vi "SetupTest.vi"(11 "Python version":string="3.9") -> ()   [LabVIEW 2020]
panel:
  in  "stop":bool
  out "Console":string
  in  "Raspberry Pi":T1={"IP Address"="raspberrypi.local", "Username"="pi", "password"="raspberry"}
  # "1. Mac Users - you might have to install commandline tools by typing xcode-select --install into the terminal and saying \"ok\"\n2. Now install paramiko - sudo -H pip3 install paramiko --ignore-installed\n3. Now install scp - sudo pip3 install scp\n4. Getting the IP address and setting up the SDCard\n     1.  https://www.raspberrypi.org/documentation/configuration/wireless/headless.md - get it on the WiFi\n     2.  https://www.raspberrypi.org/documentation/remote-access/ssh/README.md - step 3 for headless - enable SSH\n     3. https://www.raspberrypi.org/documentation/remote-access/ip-address.md to get IP address\n     3. https://www.raspberrypi.org/documentation/remote-access/ssh/unix.md - test out ssh\n5. Ping it  - ping raspberrypi.local - that will give you the IP Address\n6. SSH in\n7. Change your password"
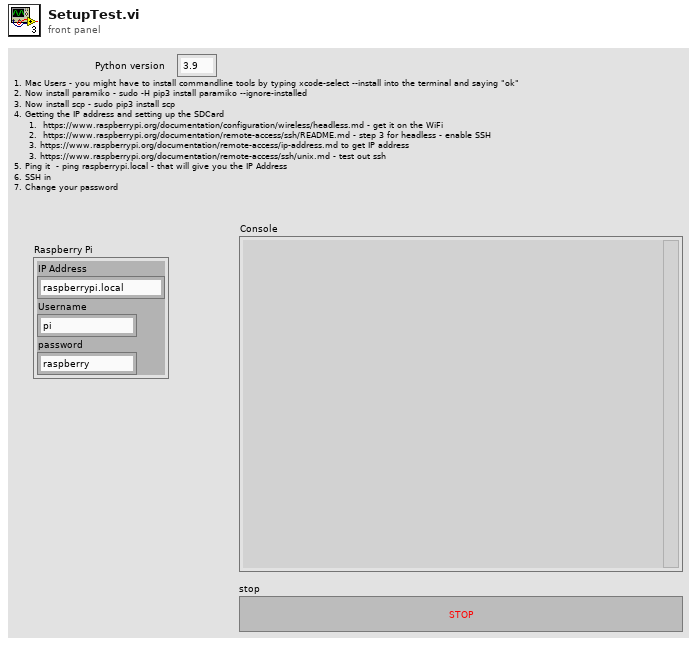
[diagram p1: front panel]
types:
  T1 = cluster{"IP Address":string, "Username":string, "password":string}
  T2 = typedef "PythonCtrl.ctl" = cluster{"session":refnum<k35>, "PyPath":path}
  T3 = typedef "eventvkey.ctl" = enum16{"ASCII", "Enter", "Return", "Shift", "Ctrl", "Alt", "Cmd", "Opt", "Caps", "NumLock", "Clear", "Break", "Up", "Down", "Left", "Right", "Insert", "Delete", "Home", "End", "PageUp", "PageDown", "Escape", "Help", "Pause", "ScrollLock", "F1", "F2", "F3", "F4", "F5", "F6", "F7", "F8", "F9", "F10", "F11", "F12", "F13", "F14", "F15", "F16", "F17", "F18", "F19", "F20", "F21", "F22", "F23", "F24", "Play", "VolumeUp", "VolumeDown", "Mute", "Two Byte Char"}
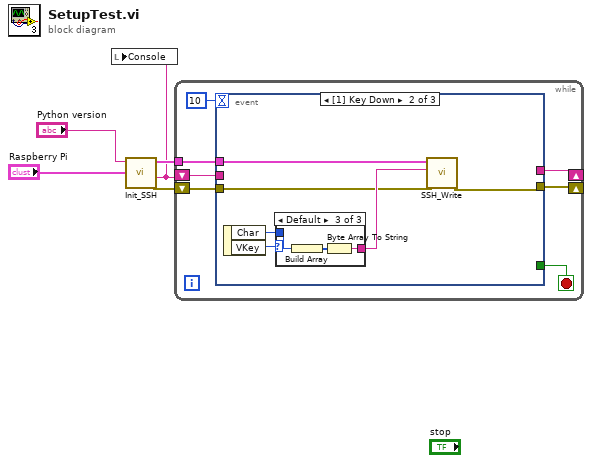
[diagram p0: block diagram]
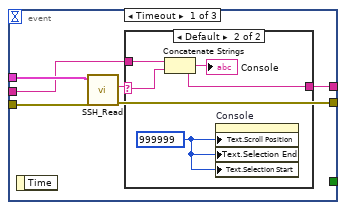
[diagram p2: hidden frame]
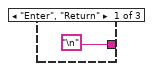
[diagram p4: hidden frame]
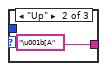
[diagram p5: hidden frame]
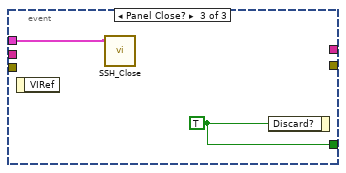
[diagram p6: hidden frame]
diagram:
  n1 = call "Init_SSH.vi"("Raspberry Pi"="Raspberry Pi", "Python version"="Python version") -> ("error out"=w2:errorcluster, "Console out"=w1:string, "Python"=w3:T2)  [unwired: 7 in]
  n2 = local write "Console"(w1) -> ()
  n3 = while {
    tunnel: w3 -> [w11]
    shift-right: [w8] -> _
    shift-left: w1 -> [w6]
    shift-right: [w7] -> _
    shift-left: w2 -> [w9]
    stop <- w12 stop-if-true
    n4 = event shown="[1] Key Down" {
      selector: _ -> [_ _ _]
      dyn-events: _ -> [_ _ _]
      timeout: 10 -> [_ _ _]
      tunnel: [_ _ w36] -> w12
      tunnel: w11 -> [w18 w27 w35]
      tunnel: w9 -> [w17 w25 _]
      tunnel: [w14 _ _] -> w8
      tunnel: [w16 w24 _] -> w7
      tunnel: w6 -> [w15 _ _]
      event Timeout {
        n5 = event-data() -> ()  [unwired: 1 in, 1 out]
        n6 = call "SSH_Read.vi"("error in (no error)"=w17, "Python"=w18) -> ("error out"=w16:errorcluster, "Reply"=w13:string)  [unwired: 7 in, 1 out]
        n7 = case shown="Default" w13 {
          selector: w13 -> [_ w20]
          tunnel: w15 -> [w19 w23]
          tunnel: [w19 w22] -> w14
          frame "" {
          }
          frame Default {
            w21 = u32 999999 ("Text.Scroll Position")
            n8 = Concatenate Strings(w23, w20) -> (w22:string)
            "Console" <- w22
            n9 = property on="Console" class="Str"("Text.Scroll Position"=w21, "Text.Selection End"=w21, "Text.Selection Start"=w21) -> ()  [unwired: 2 in, 2 out]
          }
        }
      }
      event Key Down {
        n10 = event-data() -> ("Char"=w29:i16, "VKey"=w28:T3)  [unwired: 1 in]
        n11 = case shown="Default" w28 {
          tunnel: w29 -> [_ _ w34]
          tunnel: ["\n" ("replace string (\"\")") "\u001b[A" ("replace string (\"\")") w32] -> w26
          frame "Enter", "Return" {
          }
          frame "Up" {
          }
          frame Default {
            n12 = Build Array(w34) -> (w33:i16[])
            n13 = Byte Array To String(unsigned byte array=w33) -> (string=w32:string)
          }
        }
        n14 = call "SSH_Write.vi"("error in (no error)"=w25, "Text to write"=w26, "Python in"=w27) -> ("error out"=w24:errorcluster)  [unwired: 7 in, 1 out]
      }
      event Panel Close? {
        w36 = TRUE ("Discard?")
        n15 = event-data() -> ()  [unwired: 1 in, 1 out]
        n16 = call "SSH_Close.vi"("Python"=w35) -> ()  [unwired: 11 in]
        n17 = event-data("Discard?"=w36) -> ()  [unwired: 1 in, 1 out]
      }
    }
  }
